vi "Post-Init.vi"(8 "error in (no error)":errorcluster, 11 "RP I-V Driver in":refnum<class "RP I-V Driver.lvclass">) -> (0 "error out":errorcluster, 2 "Init Result":refnum<class "Acquired Result.lvclass">, 3 "RP I-V Driver out":refnum<class "RP I-V Driver.lvclass">)   [LabVIEW 2016, in "RP I-V Driver.lvclass"]
uses:
  RP I-V Driver.lvclass
  C:/github/NHMFL_Core/Libraries/Instruments/Pulse Driver/Pulse Driver.lvclass
  Instruments/Results/Acquired Result/Acquired Result.lvclass
  Instruments/Pulse Driver/Pulse Driver.lvclass/Pulse Driver.ctl
  Instruments/Pulse Driver/Read t0.vi
  Instruments/Pulse Driver/Write t0.vi
  Red Pitaya Digitizer/Red Pitaya Digitizer.lvclass
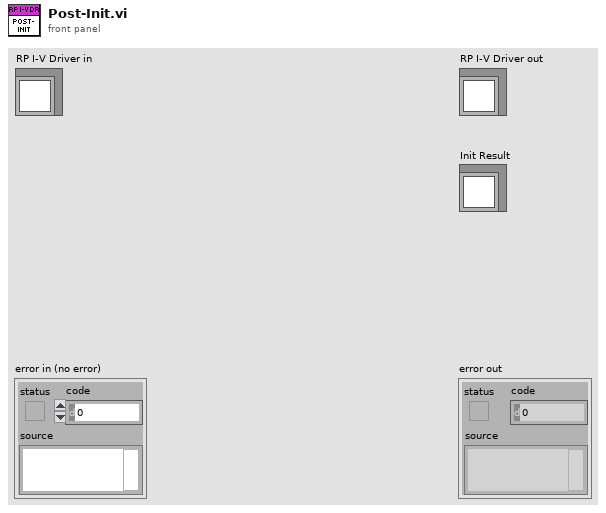
[diagram p1: front panel]
types:
  T1 = typedef "RP I-V Configuration.ctl" = cluster{"I-V parameters":T2, "Ranges":dbl[], "Pre-trigger duration":dbl, "Post-trigger duration":dbl, "Output delay":dbl}
  T2 = typedef "I-V parameters.ctl" = cluster{"Start magnitude":dbl, "Magnitude increment":dbl, "End magnitude":dbl, "Ramp length":i32, "Top  length":i32, "Threshold ":dbl, "Processing delay":u16, "Valhalla range":dbl, "Interpolation":i32, "Stop after":u16, "Detector window":i32}
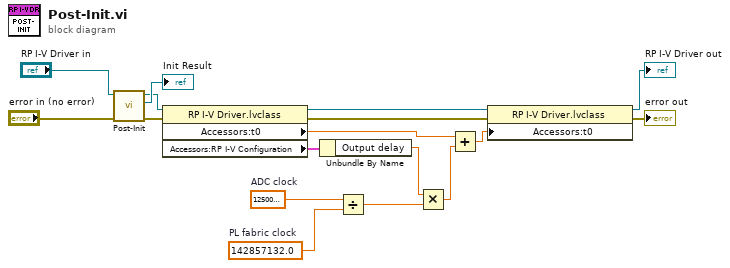
[diagram p0: block diagram]
diagram:
  w5 = 125000000.0  # ADC clock
  w4 = 142857132.0  # PL fabric clock
  n1 = call-parent "Post-Init.vi"("error in (no error)"="error in (no error)", "Pulse Driver in"="RP I-V Driver in") -> ("error out"=w17:errorcluster, "Init Result"=→"Init Result":refnum<class "Acquired Result.lvclass">, "Pulse Driver out"=w12:refnum<class "RP I-V Driver.lvclass">)  [unwired: 7 in]
  n2 = property class="RP I-V Driver.lvclass"(reference=w12, error in=w17) -> (reference out=w10:refnum<class "RP I-V Driver.lvclass">, error out=w13:errorcluster, "Accessors:t0"=w7:dbl, "Accessors:RP I-V Configuration"=w8:T1)
  n3 = Unbundle By Name(w8) -> ("Output delay"=w1:dbl)
  n4 = Divide(x=w5, y=w4) -> (x/y=w2:dbl)
  n5 = Multiply(x=w1, y=w2) -> (x*y=w3:dbl)
  n6 = Add(x=w7, y=w3) -> (x+y=w6:dbl)
  n7 = property class="RP I-V Driver.lvclass"(reference=w10, error in=w13, "Accessors:t0"=w6) -> (reference out=→"RP I-V Driver out":refnum<class "RP I-V Driver.lvclass">, error out=→"error out":errorcluster)
